vi "Report Write RES Data.vi"(8 "error in (no error)":errorcluster, 10 "report in":refnum<class "NI_report.lvclass">, 11 "Hardware Resources in":T1={"Test Setting"={"Test_Num"=0, "Test_ID"=0, "Proc_ID"=0, "Max Force"=0.0, "User"="", "SN"="", "Date"=""}, "Measurements"=[[""]], "LOG REF"=refnum, "Report Template"=path "", "Save Report path"=path "", "Data File Path"=path "", "Popup Dialog"=FALSE}) -> (0 "error out":errorcluster, 2 "report out":refnum<class "NI_report.lvclass">, 3 "Hardware Resources out":T1)   [LabVIEW 2020, in "Report.lvlib"]
doc: "Perform the acquisition. Replace the contents of this diagram with calls to acquisition hardware."
uses:
  Report.lvlib
  REP Configuration.ctl
  Test Setting.ctl
  <vilib>/Utility/NIReport.llb/NI_report.lvclass
  <vilib>/addons/_office/excel.llb/Excel Easy Table (str).vi
  <vilib>/addons/_office/NI_ReportGenerationToolkit.lvlib
  <vilib>/Utility/NIReport.llb/Excel/NI_Excel.lvclass
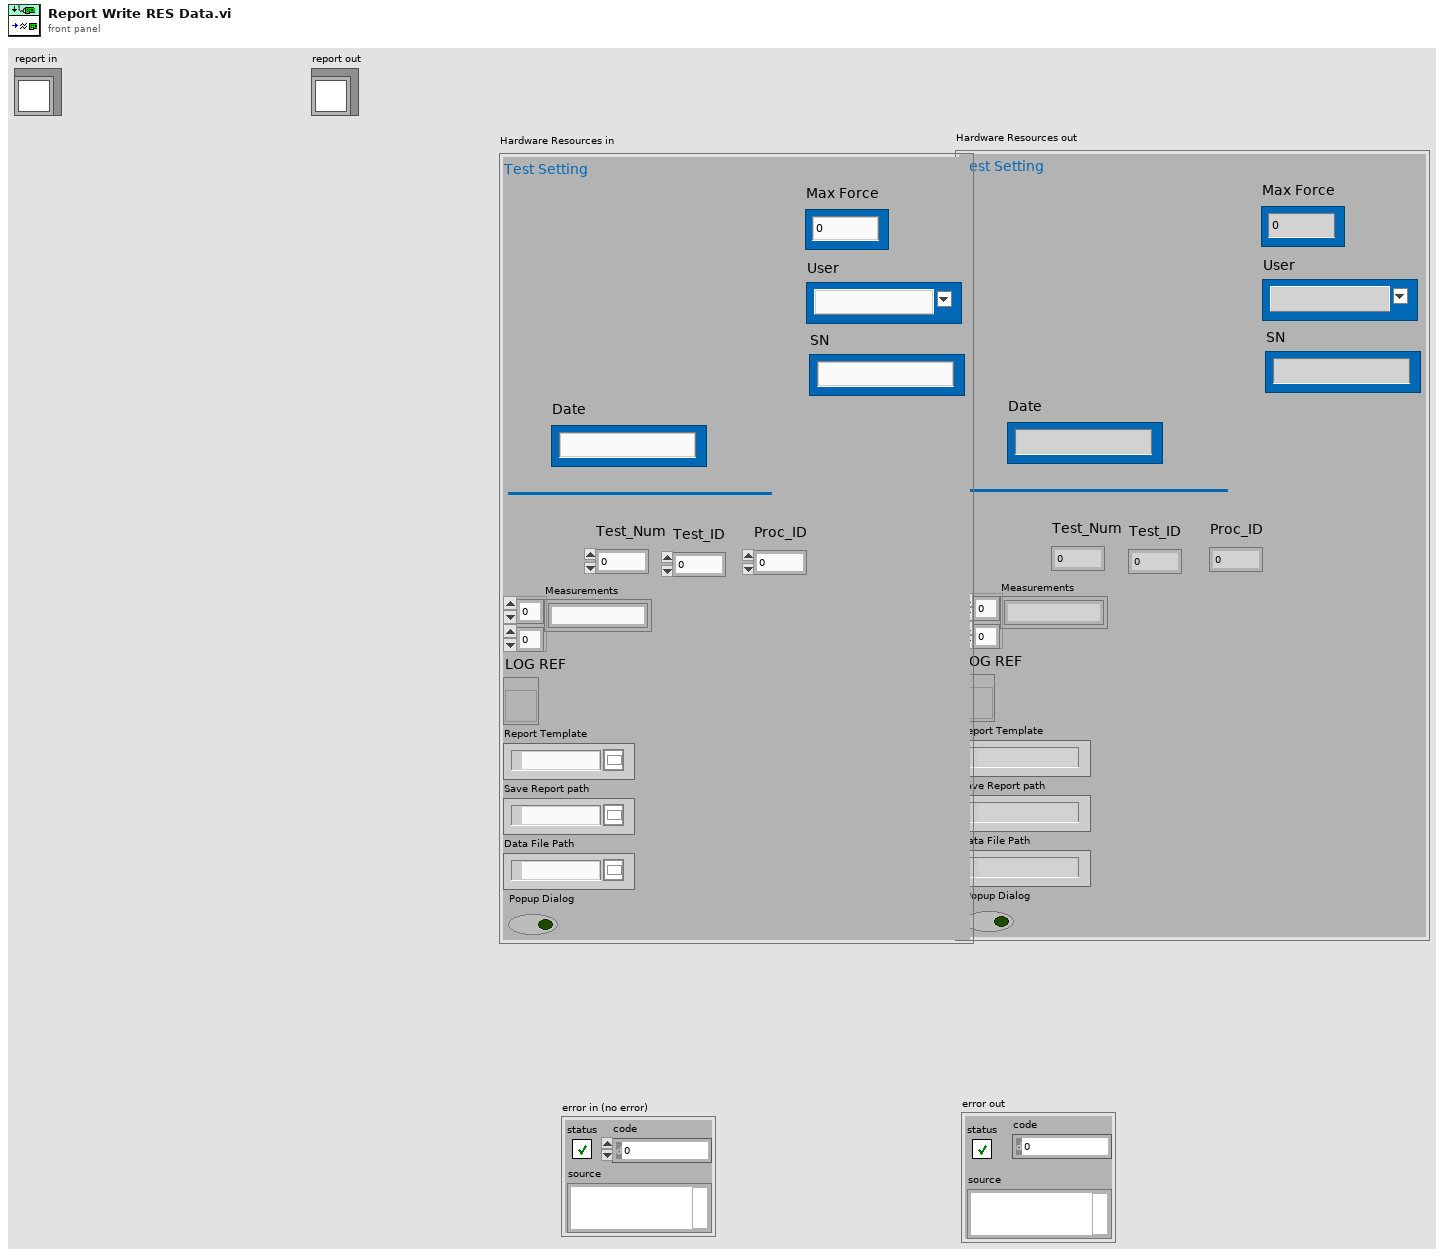
[diagram p1: front panel]
types:
  T1 = typedef "Report.lvlib/REP Configuration.ctl" = cluster{"Test Setting":T2, "Measurements":string[][], "LOG REF":refnum<vi>, "Report Template":path, "Save Report path":path, "Data File Path":path, "Popup Dialog":bool}
  T2 = typedef "Report.lvlib/Test Setting.ctl" = cluster{"Test_Num":i32, "Test_ID":i32, "Proc_ID":i32, "Max Force":dbl, "User":string, "SN":string, "Date":string}
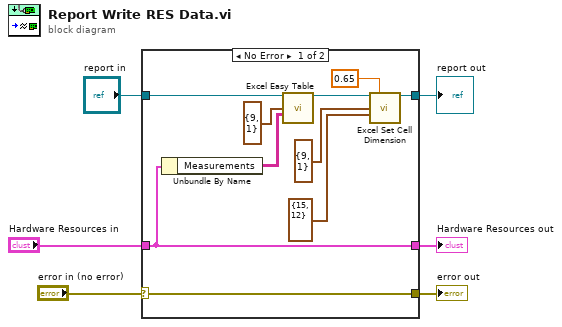
[diagram p0: block diagram]
diagram:
  n1 = case shown="No Error" "error in (no error)" {
    selector: "error in (no error)" -> [w16 w18]
    tunnel: [w16 w18] -> w5
    tunnel: "Hardware Resources in" -> [w15 w19]
    tunnel: [w15 w19] -> w3
    tunnel: "report in" -> [w14 w17]
    tunnel: [w11 w17] -> w1
    frame No Error {
      n2 = Unbundle By Name(w15) -> ("Measurements"=w7:string[][])
      n3 = call-poly <vilib>:"Excel Easy Table.vi"("report in"=w14, "start (0, 0)"=cluster{"row":i32, "column":i32} {"row"=9, "column"=1}, "text data"=w7) -> ("report out"=w12:refnum<class "NI_report.lvclass">)  [unwired: 8 in, 4 out]
      n4 = call <vilib>:"Excel Set Cell Dimension.vi"("report in"=w12, "width (-1)"=0.65, "start (-1, -1)"=cluster{"row":i32, "column":i32} {"row"=9, "column"=1} ("start (0, 0)"), "end (-1, -1)"=cluster{"row":i32, "column":i32} {"row"=15, "column"=12} ("start (0, 0)")) -> ("report out"=w11:refnum<class "NI_report.lvclass">)  [unwired: 10 in, 1 out]
    }
    frame Error {
    }
  }
  "Hardware Resources out" <- w3
  "error out" <- w5
  "report out" <- w1
